vi "Terminal-PressureSystem-LubricateUnit-Getter.vi"(8 "error in (no error)":errorcluster caption="错误输入（无错误）", 11 "read operation timeout (ms)":i32=5000 caption="读操作超时（5000毫秒）") -> (0 "error out":errorcluster caption="错误输出", 2 "时间标识":timestamp, 3 "液压子系统试验轴承润滑单元":T1)   [LabVIEW 2014]
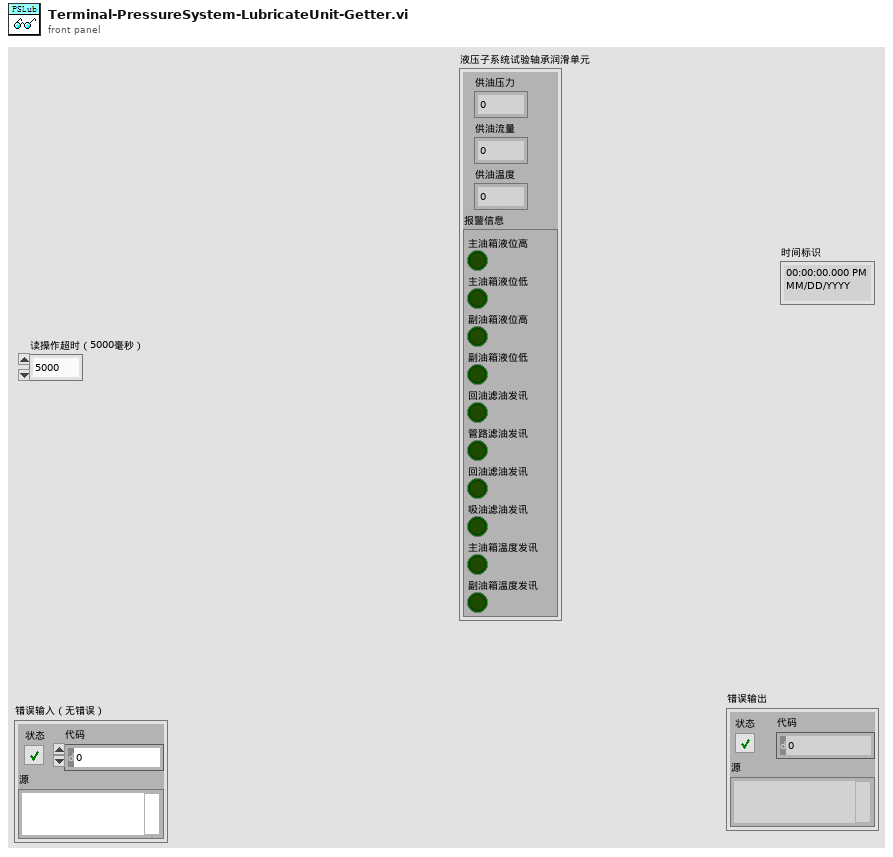
[diagram p1: front panel]
types:
  T1 = cluster{"供油压力":u16, "供油流量":u16, "供油温度":u16, "报警信息":cluster{"主油箱液位高":bool, "主油箱液位低":bool, "副油箱液位高":bool, "副油箱液位低":bool, "回油滤油发讯":bool, "管路滤油发讯":bool, "回油滤油发讯":bool, "吸油滤油发讯":bool, "主油箱温度发讯":bool, "副油箱温度发讯":bool}}
  T2 = cluster{"主油箱液位高":bool, "主油箱液位低":bool, "副油箱液位高":bool, "副油箱液位低":bool, "回油滤油发讯":bool, "管路滤油发讯":bool, "回油滤油发讯":bool, "吸油滤油发讯":bool, "主油箱温度发讯":bool, "副油箱温度发讯":bool}
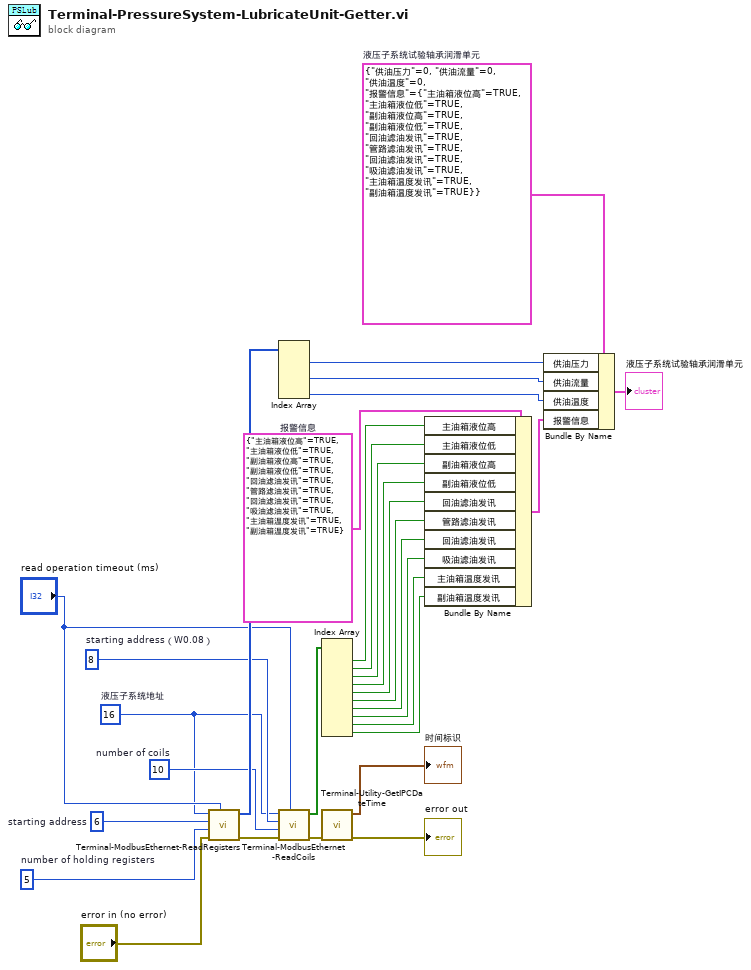
[diagram p0: block diagram]
diagram:
  w14 = T2 {"主油箱液位高"=TRUE, "主油箱液位低"=TRUE, "副油箱液位高"=TRUE, "副油箱液位低"=TRUE, "回油滤油发讯"=TRUE, "管路滤油发讯"=TRUE, "回油滤油发讯"=TRUE, "吸油滤油发讯"=TRUE, "主油箱温度发讯"=TRUE, "副油箱温度发讯"=TRUE}  # 报警信息
  w21 = u16 10  # number of coils
  w22 = u16 8  # starting address（W0.08）
  w28 = T1 {"供油压力"=0, "供油流量"=0, "供油温度"=0, "报警信息"={"主油箱液位高"=TRUE, "主油箱液位低"=TRUE, "副油箱液位高"=TRUE, "副油箱液位低"=TRUE, "回油滤油发讯"=TRUE, "管路滤油发讯"=TRUE, "回油滤油发讯"=TRUE, "吸油滤油发讯"=TRUE, "主油箱温度发讯"=TRUE, "副油箱温度发讯"=TRUE}}  # 液压子系统试验轴承润滑单元
  w10 = u16 5  # number of holding registers
  w30 = u16 6  # starting address
  w3 = u8 16  # 液压子系统地址
  n1 = call "Terminal-ModbusEthernet-ReadRegisters.vi"("read operation timeout (ms)"="read operation timeout (ms)", "error in"="error in (no error)", "number of holding registers"=w10, "starting address"=w30, "unit ID"=w3) -> ("error out"=w4:errorcluster, "register values"=w24:u16[])  [unwired: 5 in]
  n2 = Index Array(array=w24) -> (element #1=w27:u16, element #3=w2:u16, element #5=w1:u16)  [unwired: 5 in, 2 out]
  n3 = call "Terminal-ModbusEthernet-ReadCoils.vi"("read operation timeout (ms)"="read operation timeout (ms)", "error in"=w4, "number of coils"=w21, "starting address"=w22, "unit ID"=w3) -> ("error out"=w23:errorcluster, "coil values"=w20:bool[])  [unwired: 5 in]
  n4 = Index Array(array=w20) -> (element #1=w19:bool, element #2=w18:bool, element #3=w17:bool, element #4=w16:bool, element #5=w15:bool, element #6=w9:bool, element #7=w8:bool, element #8=w7:bool, element #9=w6:bool, element #10=w5:bool)  [unwired: 10 in]
  n5 = call "Terminal-Utility-GetIPCDateTime.vi"("error in (no error)"=w23) -> ("error out"=→"error out":errorcluster, "时间标识"=→"时间标识":timestamp)  [unwired: 9 in]
  n6 = Bundle By Name(cluster=w14, "主油箱液位高"=w19, "主油箱液位低"=w18, "副油箱液位高"=w17, "副油箱液位低"=w16, "回油滤油发讯"=w15, "管路滤油发讯"=w9, "回油滤油发讯"=w8, "吸油滤油发讯"=w7, "主油箱温度发讯"=w6, "副油箱温度发讯"=w5) -> (w13:T2)
  n7 = Bundle By Name(cluster=w28, "供油压力"=w27, "供油流量"=w2, "供油温度"=w1, "报警信息"=w13) -> (→"液压子系统试验轴承润滑单元":T1)
